vi "Write Address.vi"(10 "Address":string, 11 "Network Stream":refnum<class "Network Stream.lvclass">) -> (3 "Network Stream out":refnum<class "Network Stream.lvclass">)   [LabVIEW 2023, in "Network Stream.lvclass"]
uses:
  Network Stream.lvclass
  Network Stream.lvclass/Network Stream.ctl
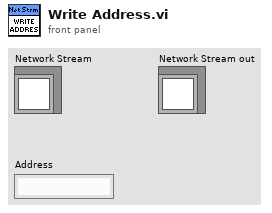
[diagram p1: front panel]
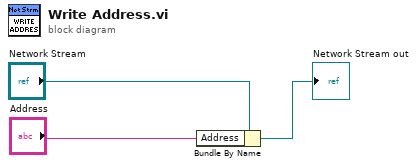
[diagram p0: block diagram]
diagram:
  n1 = Bundle By Name(cluster="Network Stream", "Address"="Address") -> (→"Network Stream out":refnum<class "Network Stream.lvclass">)
